vi "only[2][1].vi"() -> ()   [LabVIEW 2025]
panel:
  out "x = LA":bool
  out "x = RE":bool
  in  "path 13":path
  out "x = RC":bool
  in  "path 12":path
  out "x = RF":bool
  in  "path 11":path
  out "x = RD":bool
  in  "path 10":path
  out "x = RA":bool
  in  "path 9":path
  out "x = LF":bool
  in  "path 8":path
  out "x =RB":bool
  in  "path 7":path
  out "x = LG":bool
  in  "path 6":path
  out "x = LD":bool
  in  "path 5":path
  out "x =LB":bool
  in  "path 4":path
  out "x = LE":bool
  in  "path 3":path
  out "x = LC":bool
  in  "path 2":path
  out "x = RG":bool
  in  "stop":bool
  in  "path":path
  out "text":string
  in  "file (use dialog)":path
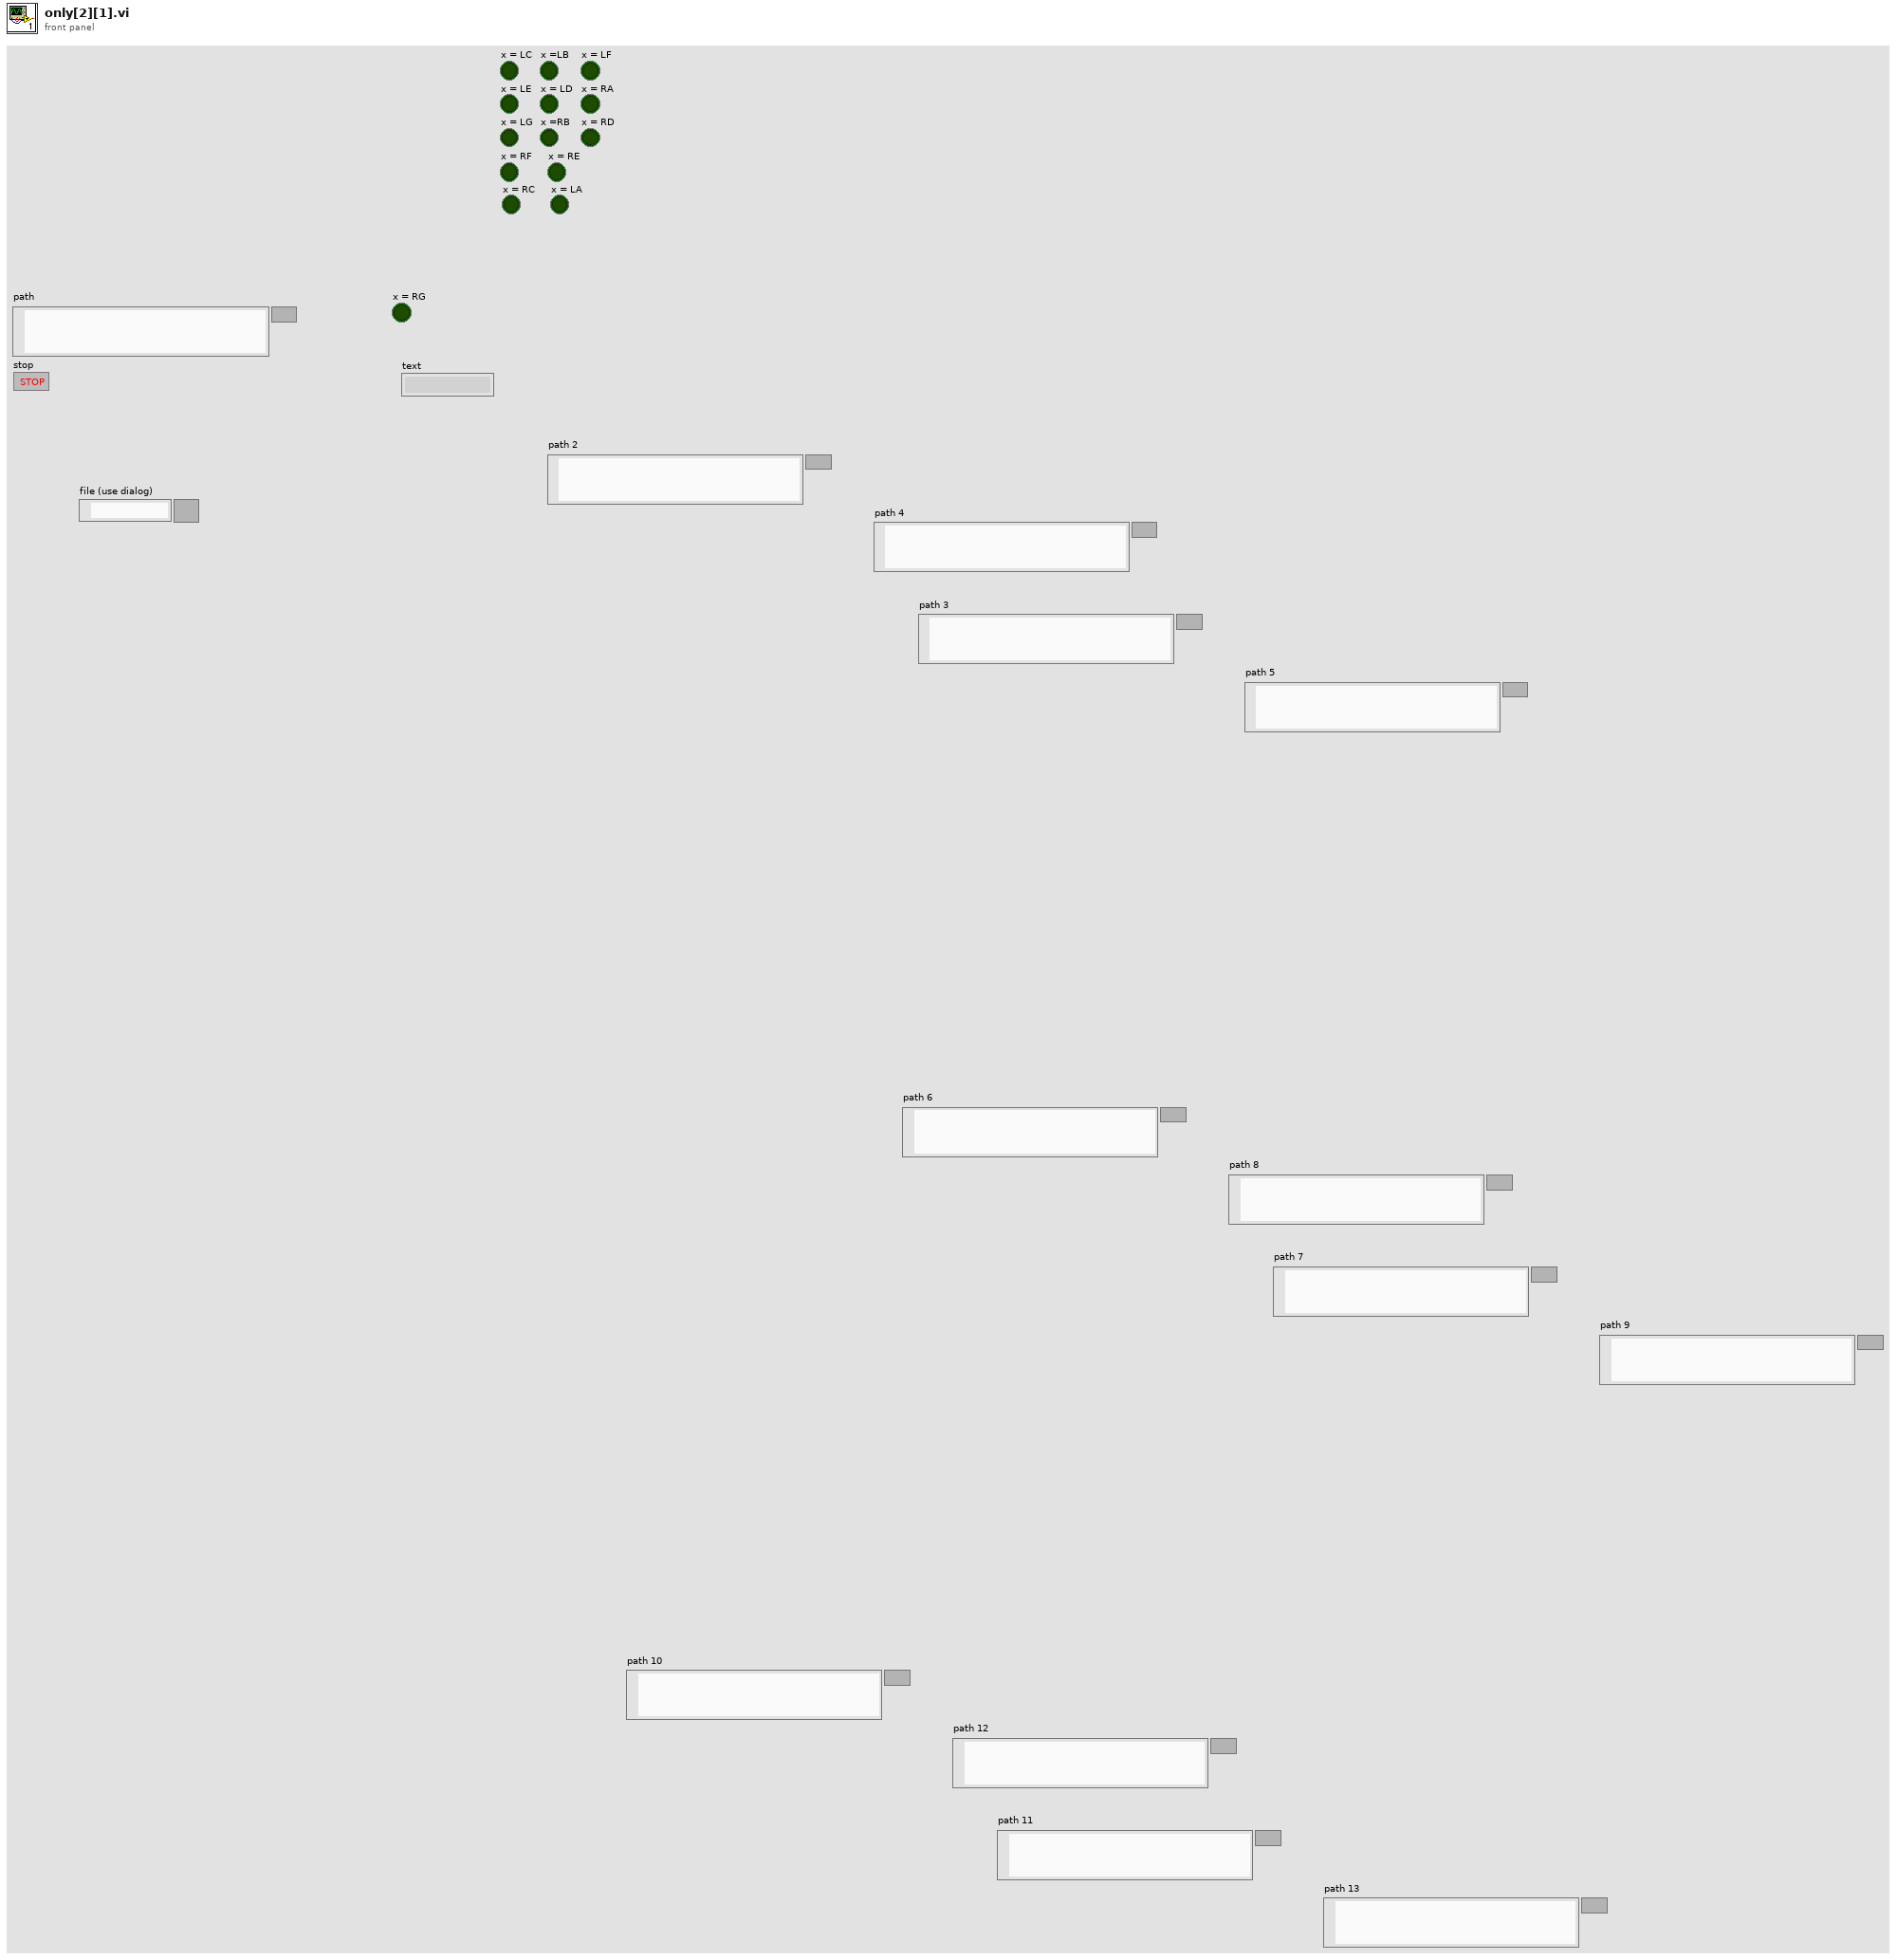
[diagram p1: front panel]
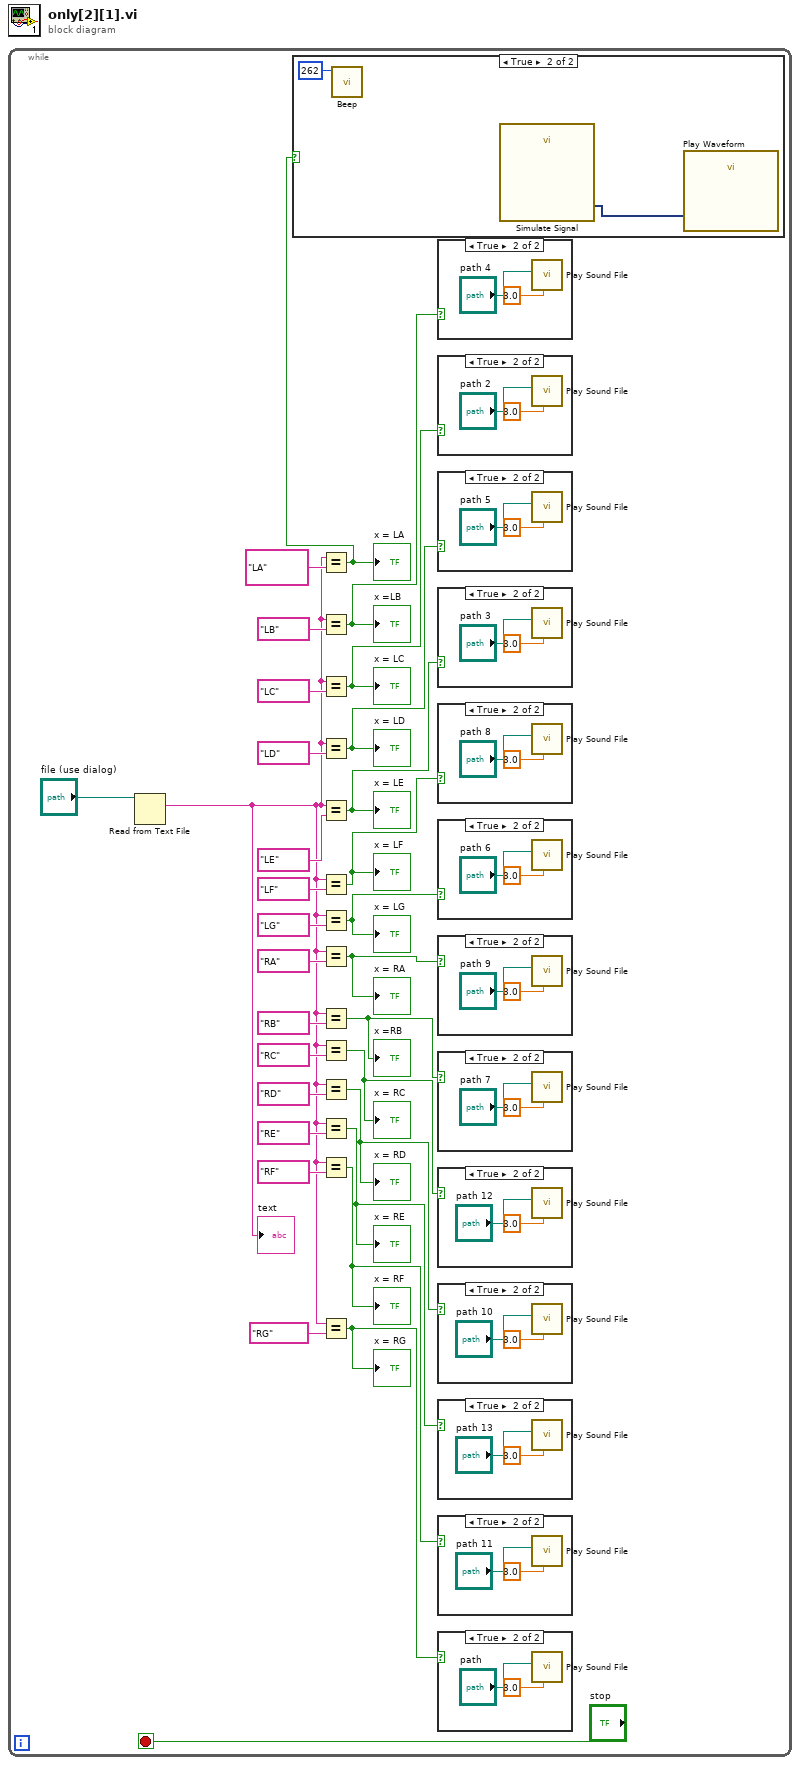
[diagram p0: block diagram]
diagram:
  n1 = while {
    stop <- "stop" stop-if-true
    n2 = Read from Text File(file (use dialog)="file (use dialog)") -> (text=w1:string)  [unwired: 3 in, 3 out]
    "text" <- w1
    n3 = Equal?(x=w1, y="LA") -> (x = y?=w2:bool)
    "x = LA" <- w2
    n4 = case shown="True" w2 {
      frame False {
      }
      frame True {
        n5 = call <vilib>:"Beep.vi"("frequency (Hz)"=u32 262) -> ()  [unwired: 11 in]
        n6 = call "Simulate Signal"() -> ("Sine"=w32:dynamicdata)  [unwired: 14 in, 1 out]
        n7 = call "Play Waveform"("Data"=w32) -> ()  [unwired: 18 in, 1 out]
      }
    }
    n8 = Equal?(x=w1, y="LB") -> (x = y?=w22:bool)
    "x =LB" <- w22
    n9 = Equal?(x=w1, y="LC") -> (x = y?=w26:bool)
    "x = LC" <- w26
    n10 = Equal?(x=w1, y="LD") -> (x = y?=w20:bool)
    "x = LD" <- w20
    n11 = Equal?(x=w1, y="LE") -> (x = y?=w24:bool)
    "x = LE" <- w24
    n12 = Equal?(x=w1, y="LF") -> (x = y?=w14:bool)
    "x = LF" <- w14
    n13 = Equal?(x=w1, y="LG") -> (x = y?=w18:bool)
    "x = LG" <- w18
    n14 = Equal?(x=w1, y="RA") -> (x = y?=w12:bool)
    "x = RA" <- w12
    n15 = Equal?(x=w1, y="RB") -> (x = y?=w16:bool)
    "x =RB" <- w16
    n16 = Equal?(x=w1, y="RC") -> (x = y?=w6:bool)
    "x = RC" <- w6
    n17 = Equal?(x=w1, y="RD") -> (x = y?=w10:bool)
    "x = RD" <- w10
    n18 = Equal?(x=w1, y="RE") -> (x = y?=w4:bool)
    "x = RE" <- w4
    n19 = Equal?(x=w1, y="RF") -> (x = y?=w8:bool)
    "x = RF" <- w8
    n20 = Equal?(x=w1, y="RG") -> (x = y?=w29:bool)
    "x = RG" <- w29
    n21 = case shown="True" w22 {
      frame False {
      }
      frame True {
        n22 = call <vilib>:"Play Sound File.vi"("timeout (sec)"=3.0, "path"="path 4") -> ()  [unwired: 8 in, 2 out]
      }
    }
    n23 = case shown="True" w26 {
      frame False {
      }
      frame True {
        n24 = call <vilib>:"Play Sound File.vi"("timeout (sec)"=3.0, "path"="path 2") -> ()  [unwired: 8 in, 2 out]
      }
    }
    n25 = case shown="True" w20 {
      frame False {
      }
      frame True {
        n26 = call <vilib>:"Play Sound File.vi"("timeout (sec)"=3.0, "path"="path 5") -> ()  [unwired: 8 in, 2 out]
      }
    }
    n27 = case shown="True" w24 {
      frame False {
      }
      frame True {
        n28 = call <vilib>:"Play Sound File.vi"("timeout (sec)"=3.0, "path"="path 3") -> ()  [unwired: 8 in, 2 out]
      }
    }
    n29 = case shown="True" w14 {
      frame False {
      }
      frame True {
        n30 = call <vilib>:"Play Sound File.vi"("timeout (sec)"=3.0, "path"="path 8") -> ()  [unwired: 8 in, 2 out]
      }
    }
    n31 = case shown="True" w18 {
      frame False {
      }
      frame True {
        n32 = call <vilib>:"Play Sound File.vi"("timeout (sec)"=3.0, "path"="path 6") -> ()  [unwired: 8 in, 2 out]
      }
    }
    n33 = case shown="True" w12 {
      frame False {
      }
      frame True {
        n34 = call <vilib>:"Play Sound File.vi"("timeout (sec)"=3.0, "path"="path 9") -> ()  [unwired: 8 in, 2 out]
      }
    }
    n35 = case shown="True" w16 {
      frame False {
      }
      frame True {
        n36 = call <vilib>:"Play Sound File.vi"("timeout (sec)"=3.0, "path"="path 7") -> ()  [unwired: 8 in, 2 out]
      }
    }
    n37 = case shown="True" w6 {
      frame False {
      }
      frame True {
        n38 = call <vilib>:"Play Sound File.vi"("timeout (sec)"=3.0, "path"="path 12") -> ()  [unwired: 8 in, 2 out]
      }
    }
    n39 = case shown="True" w10 {
      frame False {
      }
      frame True {
        n40 = call <vilib>:"Play Sound File.vi"("timeout (sec)"=3.0, "path"="path 10") -> ()  [unwired: 8 in, 2 out]
      }
    }
    n41 = case shown="True" w4 {
      frame False {
      }
      frame True {
        n42 = call <vilib>:"Play Sound File.vi"("timeout (sec)"=3.0, "path"="path 13") -> ()  [unwired: 8 in, 2 out]
      }
    }
    n43 = case shown="True" w8 {
      frame False {
      }
      frame True {
        n44 = call <vilib>:"Play Sound File.vi"("timeout (sec)"=3.0, "path"="path 11") -> ()  [unwired: 8 in, 2 out]
      }
    }
    n45 = case shown="True" w29 {
      frame False {
      }
      frame True {
        n46 = call <vilib>:"Play Sound File.vi"("timeout (sec)"=3.0, "path"="path") -> ()  [unwired: 8 in, 2 out]
      }
    }
  }
